vi "Spanbenennung Stringarray.vi"(0 "Spangaseingänge":i32, 11 "error in (no error)":errorcluster caption="Fehler (Eingang, kein Fehler)") -> (4 "Span Eingänge":string[](array[string]), 15 "error out":errorcluster caption="Fehler (Ausgang)")   [LabVIEW 2020, in "CalGas Aufschaltung.lvlib"]
uses:
  CalGas Aufschaltung.lvlib
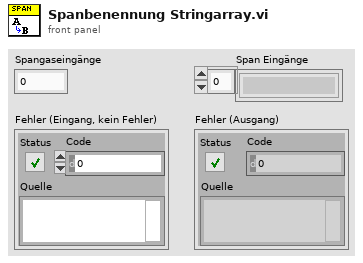
[diagram p1: front panel]
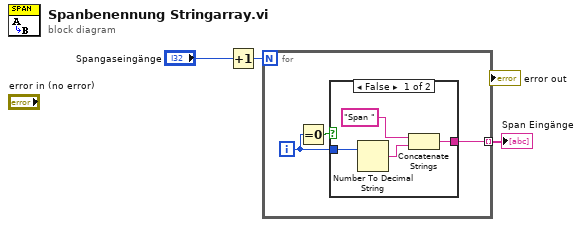
[diagram p0: block diagram]
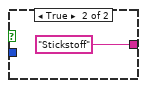
[diagram p2: hidden frame]
diagram:
  n1 = Increment(x="Spangaseingänge") -> (x+1=w2:i32)
  n2 = for {
    N: w2 -> [_]
    tunnel: [w4] -> w1 mode=indexing
    i -> [w5]
    n3 = Equal To 0?(x=w5) -> (x = 0?=w6:bool)
    n4 = case shown="False" w6 {
      tunnel: w5 -> [w8 _]
      tunnel: [w7 "Stickstoff"] -> w4
      frame False {
        n5 = Number To Decimal String(number=w8) -> (decimal integer string=w9:string)  [unwired: 1 in]
        n6 = Concatenate Strings("Span ", w9) -> (w7:string)
      }
      frame True {
      }
    }
  }
  "Span Eingänge" <- w1
